vi "SingleIV.vi"(0 "UiDefinition 2":T1) -> (4 "appended array":dbl[][](array[numeric]), 6 "CapacitanceIV":dbl, 10 "slope":dbl, 15 "intercept":dbl)   [LabVIEW 2020]
uses:
  UIReferences.ctl
  D:/LabviewDXFViewer/LabviewDXFViewer/bin/Release/LabviewDXFViewer.exe
  LabviewDXFViewer/bin/Release/LabviewDXFViewer.exe
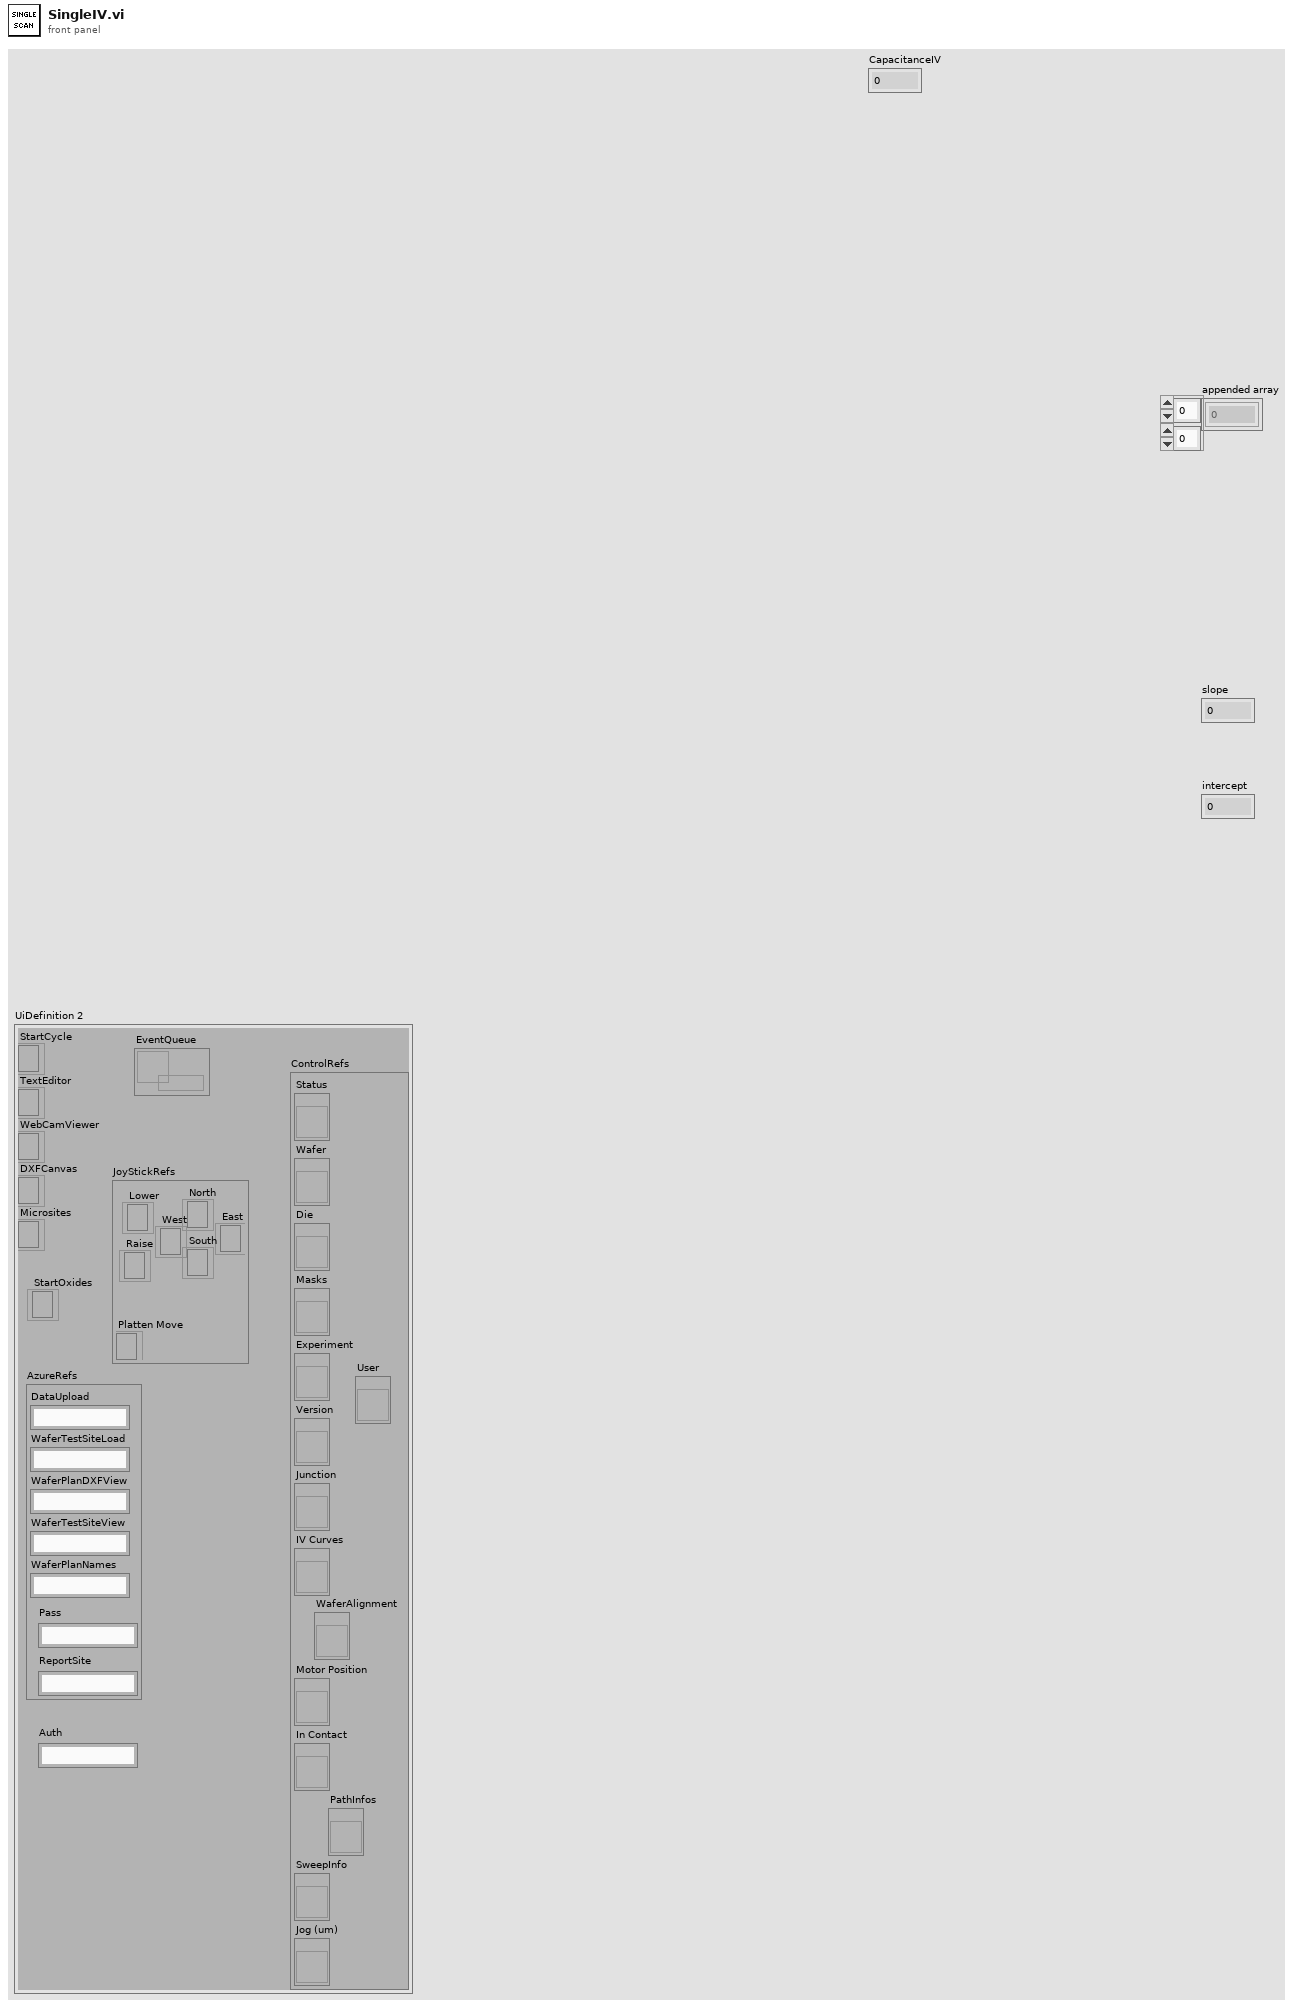
[diagram p1: front panel]
types:
  T1 = typedef "UIReferences.ctl" = cluster{"StartCycle":refnum<k24>, "TextEditor":refnum<k24>, "WebCamViewer":refnum<k24>, "DXFCanvas":refnum<k24>, "Microsites":refnum<k24>, "JoyStickRefs":cluster{"North":refnum<k24>, "Lower":refnum<k24>, "Raise":refnum<k24>, "Platten Move":refnum<k24>, "West":refnum<k24>, "East":refnum<k24>, "South":refnum<k24>}, "AzureRefs":cluster{"DataUpload":string, "WaferTestSiteLoad":string, "WaferPlanDXFView":string, "WaferTestSiteView":string, "WaferPlanNames":string, "Pass":string, "ReportSite":string}, "ControlRefs":cluster{"Status":refnum<vi>, "Wafer":refnum<vi>, "Die":refnum<vi>, "Masks":refnum<vi>, "Experiment":refnum<vi>, "Version":refnum<vi>, "Junction":refnum<vi>, "IV Curves":refnum<vi>, "Motor Position":refnum<vi>, "In Contact":refnum<vi>, "SweepInfo":refnum<vi>, "Jog (um)":refnum<vi>, "PathInfos":refnum<vi>, "User":refnum<vi>, "WaferAlignment":refnum<vi>}, "EventQueue":refnum<queue>, "StartOxides":refnum<k24>, "Auth":string}
  T2 = typedef "CapacitanceInfos.ctl" = cluster{"Conductance":dbl, "CapacitanceIV":dbl, "Intercept":dbl, "CapacitanceSW":dbl, "Sum":dbl, "CapacitanceInfos":T3[], "CapacitancePhase":dbl, "dC/dV":dbl, "Function":string, "OtherInfo":dbl[][]}
  T3 = typedef "CapacitanceRecord.ctl" = cluster{"Freq":dbl, "Vpp":dbl, "PhaseS":dbl, "Irms":dbl, "PhaseC":dbl, "Theta":dbl, "VDrive":dbl, "Capacitance":dbl, "Other":dbl}
  T4 = typedef "WaferAlignmentType.ctl" = cluster{"Wafer Units to microns":dbl, "Rotation Misalign":dbl[], "Scale Misalign":dbl, "Steps Per micron":dbl, "Position 1":i32[], "Position 2":i32[], "Lift Distance":i32, "Position 3":i32[], "Jog Height":i32}
  T5 = cluster{"Current Range":dbl, "Source Measure Unit Channel (0: Channel A)":i32, "Waveform":waveform(dbl), "VISA resource name":refnum<visa-resource-name>, "CodeText":string}
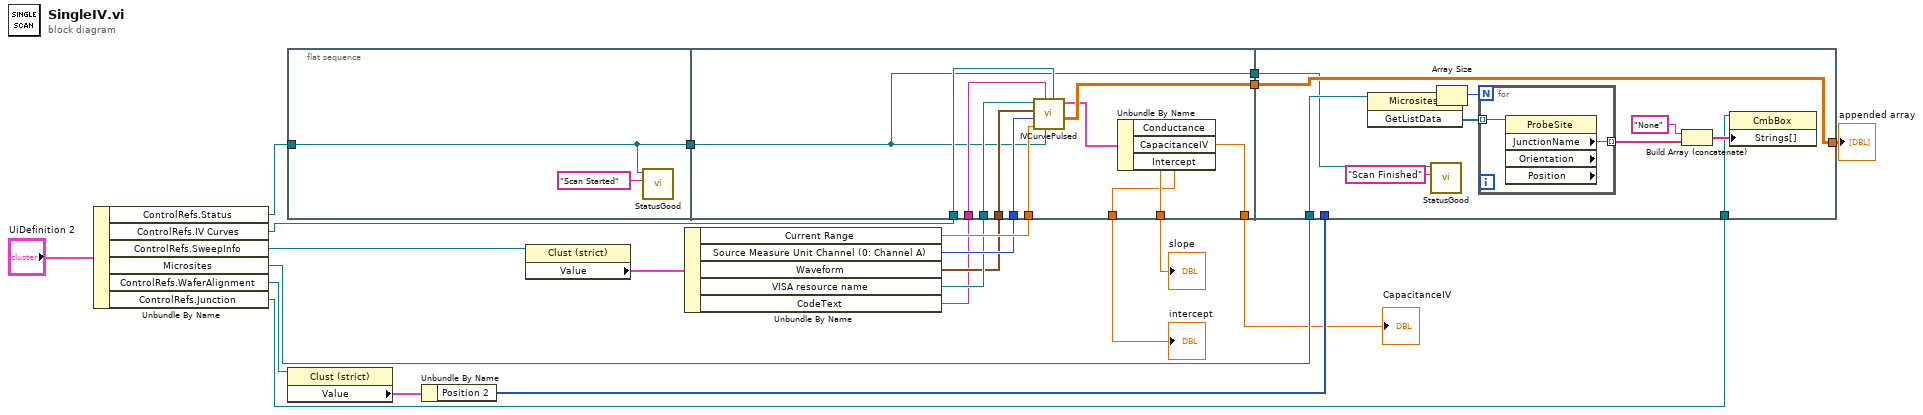
[diagram p0: block diagram]
diagram:
  n1 = Unbundle By Name("UiDefinition 2") -> ("ControlRefs.Status"=w13:refnum<vi>, "ControlRefs.IV Curves"=w12:refnum<vi>, "ControlRefs.SweepInfo"=w11:refnum<vi>, "Microsites"=w9:refnum<k24>, "ControlRefs.WaferAlignment"=w8:refnum<vi>, "ControlRefs.Junction"=w5:refnum<vi>)
  n2 = flat-sequence {
    tunnel: w13 -> [w23]
    tunnel: [w23] -> w22
    tunnel: [w36] -> w15
    tunnel: w22 -> [w25]
    tunnel: w20 -> [w35]
    tunnel: w19 -> [w34]
    tunnel: w18 -> [w33]
    tunnel: w17 -> [w32]
    tunnel: w16 -> [w31]
    tunnel: w12 -> [w30]
    tunnel: [w29] -> w4
    tunnel: [w28] -> w3
    tunnel: [w27] -> w2
    tunnel: [w25] -> w1
    tunnel: [w46] -> w21
    tunnel: w15 -> [w46]
    tunnel: w9 -> [w39]
    tunnel: w6 -> [_]
    tunnel: w5 -> [w40]
    tunnel: w1 -> [w37]
    frame #0 {
      n3 = call "StatusGood.vi"("Text.Text"="Scan Started", "String in"=w23) -> ()  [unwired: 10 in]
    }
    frame #1 {
      n4 = call "IVCurvePulsed.vi"("XYGraph Refnum"=w30, "Status"=w25, "Source Code"=w31, "CurrentRange"=w35, "Source Measure Unit Channel (0: Channel A)"=w34, "Waveform"=w32, "VISA Refnum in"=w33) -> ("appended array"=w36:dbl[][], "InfoCluster"=w26:T2)  [unwired: 3 in]
      n5 = Unbundle By Name(w26) -> ("Conductance"=w29:dbl, "CapacitanceIV"=w27:dbl, "Intercept"=w28:dbl)
    }
    frame #2 {
      n6 = invoke class="Microsites" method="GetListData"(reference=w39) -> ("GetListData"=w45:refnum<k24>[])  [unwired: 2 in, 2 out]
      n7 = call "StatusGood.vi"("Text.Text"="Scan Finished", "String in"=w37) -> ()  [unwired: 10 in]
      n8 = Array Size(array=w45) -> (size(s)=w44:i32)
      n9 = for {
        N: w44 -> [_]
        tunnel: w45 -> [w48] mode=indexing
        tunnel: [w47] -> w43 mode=indexing
        n10 = property class="ProbeSite" props=["JunctionName", "Orientation", "Position"](reference=w48) -> ("JunctionName"=w47:string)  [unwired: 1 in, 4 out]
      }
      n11 = Build Array (concatenate)("None", w43) -> (w41:string[])
      n12 = property class="CmbBox"(reference=w40, "Strings[]"=w41) -> ()  [unwired: 1 in, 2 out]
    }
  }
  n13 = property class="Clust (strict)"(reference=w8) -> ("Value"=w7:T4)  [unwired: 1 in, 2 out]
  n14 = Unbundle By Name(w7) -> ("Position 2"=w6:i32[])
  n15 = property class="Clust (strict)"(reference=w11) -> ("Value"=w10:T5)  [unwired: 1 in, 2 out]
  n16 = Unbundle By Name(w10) -> ("Current Range"=w20:dbl, "Source Measure Unit Channel (0: Channel A)"=w19:i32, "Waveform"=w17:waveform(dbl), "VISA resource name"=w18:refnum<visa-resource-name>, "CodeText"=w16:string)
  "intercept" <- w3
  "slope" <- w4
  "appended array" <- w21
  "CapacitanceIV" <- w2
